vi "Connect.vi"(0 "STOMP in":refnum<class "STOMP.lvclass">, 1 "address":string="localhost", 2 "port":u16=61613, 4 "timeout ms (60000)":i32=60000, 5 "error in":errorcluster, 7 "version":string="1.2") -> (14 "STOMP out":refnum<class "STOMP.lvclass">, 19 "error out":errorcluster)   [LabVIEW 2017, in "LabVIEW STOMP.lvlib" / "STOMP.lvclass"]
uses:
  STOMP.lvclass
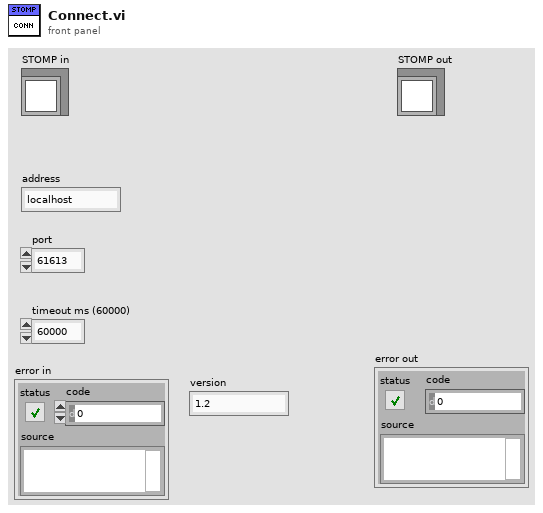
[diagram p1: front panel]
types:
  T1 = typedef "LabVIEW STOMP.lvlib/STOMP.lvclass/Type_ServerFrame.ctl" = cluster{"Type":T2, "Headers":cluster{"Header":string, "Value":string}[], "Body":string}
  T2 = typedef "LabVIEW STOMP.lvlib/STOMP.lvclass/Type_ServerFrameType.ctl" = enum16{"Undefined", "MESSAGE", "CONNECTED", "RECEIPT", "ERROR"}
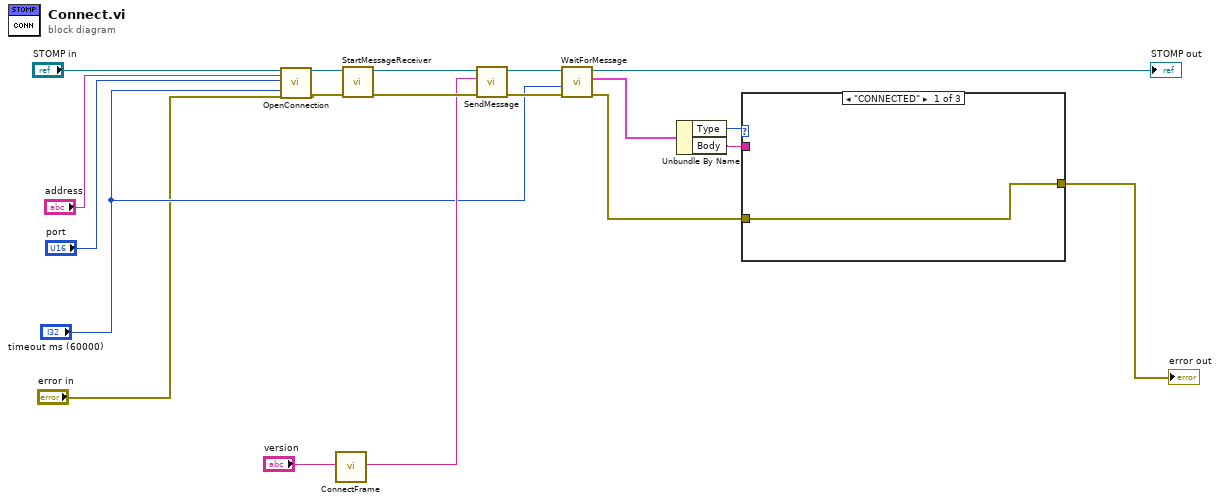
[diagram p0: block diagram]
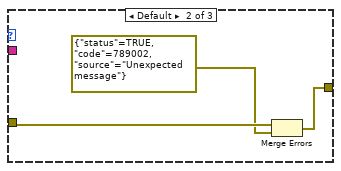
[diagram p2: hidden frame]
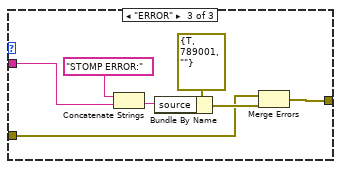
[diagram p3: hidden frame]
diagram:
  n1 = call-dynamic "OpenConnection.vi"("STOMP in"="STOMP in", "address"="address", "port"="port", "timeout ms (60000)"="timeout ms (60000)", "error in (no error)"="error in") -> ("STOMP out"=w16:refnum<class "STOMP.lvclass">, "error out"=w15:errorcluster)  [unwired: 13 in]
  n2 = call "ConnectFrame.vi"("version"="version") -> ("Connect Frame"=w10:string)  [unwired: 18 in]
  n3 = call-dynamic "StartMessageReceiver.vi"("error in (no error)"=w15, "STOMP in"=w16) -> ("error out"=w14:errorcluster, "STOMP out"=w13:refnum<class "STOMP.lvclass">)  [unwired: 8 in]
  n4 = call-dynamic "SendMessage.vi"("error in (no error)"=w14, "data in"=w10, "STOMP in"=w13) -> ("error out"=w11:errorcluster, "STOMP out"=w12:refnum<class "STOMP.lvclass">)  [unwired: 7 in]
  n5 = call-dynamic "WaitForMessage.vi"("error in (no error)"=w11, "timeout in ms (10000)"="timeout ms (60000)", "STOMP in"=w12) -> ("error out"=w1:errorcluster, "message"=w2:T1, "STOMP out"=→"STOMP out":refnum<class "STOMP.lvclass">)  [unwired: 6 in]
  n6 = Unbundle By Name(w2) -> ("Type"=w7:T2, "Body"=w6:string)
  n7 = case shown="\"CONNECTED\"" w7 {
    tunnel: w6 -> [_ _ w29]
    tunnel: w1 -> [w20 w23 w27]
    tunnel: [w20 w21 w26] -> w5
    frame "CONNECTED" {
    }
    frame Default {
      n8 = Merge Errors(w23, errorcluster {"status"=TRUE, "code"=789002, "source"="Unexpected message"} ("error constant")) -> (w21:errorcluster)
    }
    frame "ERROR" {
      n9 = Concatenate Strings("STOMP ERROR:" ("string"), w29) -> (w25:string)
      n10 = Bundle By Name(cluster=errorcluster {"status"=TRUE, "code"=789001, "source"=""} ("error constant"), "source"=w25) -> (w28:errorcluster)
      n11 = Merge Errors(w27, w28) -> (w26:errorcluster)
    }
  }
  "error out" <- w5
